vi "encodeFloat.vi"(8 "error in (no error)":errorcluster, 10 "Variant":variant) -> (0 "error out":errorcluster, 2 "Array":u8[](array[numeric]) format="%.0x")   [LabVIEW 2016, in "MsgPack.lvlib"]
uses:
  MsgPack.lvlib
  <vilib>/Utility/Data Type/NI_Data Type.lvlib
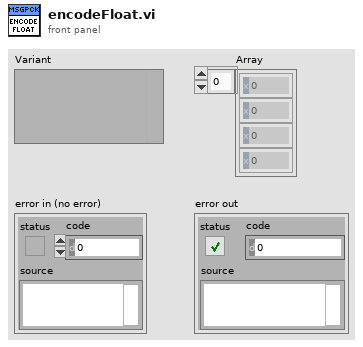
[diagram p1: front panel]
types:
  T1 = typedef "NI_Data Type.lvlib/Data Type.ctl" = enum8{"Invalid Type", "Void", "I8", "I16", "I32", "I64", "U8", "U16", "U32", "U64", "Single Float", "Double Float", "Extended Float", "Single Complex", "Double Complex", "Extended Complex", "Enum U8", "Enum U16", "Enum U32", "Enum U64", "Single Float With Unit", "Double Float With Unit", "Extended Float With Unit", "Single Complex with Unit", "Double Complex with Unit", "Extended Complex with Unit", "Boolean", "String", "Path", "Picture", "Tag", "Array", "Cluster", "Variant", "LV Variant", "Waveform", "Timestamp", "Digital Waveform", "Digital Data", "ExpressData", "Refnum", "External Data", "VI", "Poly VI", "LabVIEW Class Instance", "Fixed Point"}
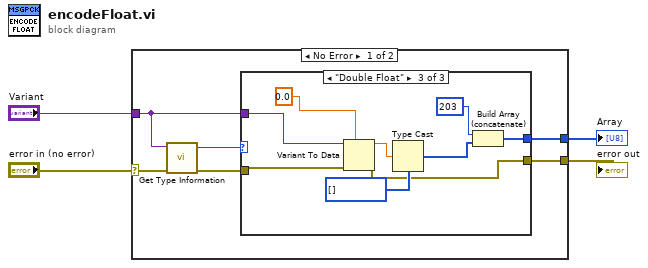
[diagram p0: block diagram]
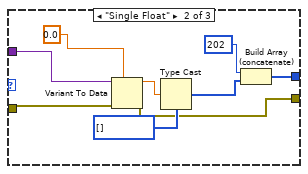
[diagram p3: hidden frame]
diagram:
  n1 = case shown="No Error" "error in (no error)" {
    selector: "error in (no error)" -> [w5 w30]
    tunnel: "Variant" -> [w8 _]
    tunnel: [w7 _] -> w3
    tunnel: [w6 w30] -> w2
    frame No Error {
      n2 = call <vilib>:"Get Type Information.vi"("error in (no error)"=w5, "Variant"=w8) -> ("error out"=w9:errorcluster, "Type"=w10:T1)  [unwired: 5 in, 3 out]
      n3 = case shown="\"Double Float\"" w10 {
        tunnel: w9 -> [w11 w20 w29]
        tunnel: w8 -> [_ w19 w28]
        tunnel: [_ w14 w23] -> w7
        tunnel: [w11 w13 w22] -> w6
        frame "Invalid Type", Default {
        }
        frame "Single Float" {
          n4 = Variant To Data(error in=w20, type=sgl 0.0, Variant=w19) -> (data=w17:sgl, error out=w13:errorcluster)
          n5 = Type Cast(type=u8[] [], x=w17) -> (*(type *) &x=w15:u8[])
          n6 = Build Array (concatenate)(u8 202, w15) -> (w14:u8[])
        }
        frame "Double Float" {
          n7 = Variant To Data(error in=w29, type=0.0, Variant=w28) -> (data=w26:dbl, error out=w22:errorcluster)
          n8 = Type Cast(type=u8[] [], x=w26) -> (*(type *) &x=w24:u8[])
          n9 = Build Array (concatenate)(u8 203, w24) -> (w23:u8[])
        }
      }
    }
    frame Error {
    }
  }
  "Array" <- w3
  "error out" <- w2
